vi "SPIM.vi"() -> ()   [LabVIEW 2015]
uses:
  Camera Properties.ctl
  Microscope Settings.ctl
  CameraState.ctl
  ModeEnum.ctl
  CameraControlTypeDef.ctl
  Stack Track.ctl
  Stack_State.ctl
  <vilib>/DAQmx/write.llb/DAQmx Write (Digital 1D Wfm NChan NSamp).vi
  <vilib>/DAQmx/write.llb/DAQmx Write (Analog 1D Wfm NChan NSamp).vi
  <vilib>/DAQmx/create/channels.llb/DAQmx Create Channel (DO-Digital Output).vi
  <vilib>/DAQmx/create/channels.llb/DAQmx Create Channel (AO-Voltage-Basic).vi
  <vilib>/Waveform/DWDTOps.llb/DWDT Append Digital Samples.vi
  <vilib>/Waveform/WDTOps.llb/WDT Append Waveforms DBL.vi
  <vilib>/Waveform/WDTOps.llb/WDT Number of Waveform Samples DBL.vi
  <vilib>/DAQmx/configure/timing.llb/DAQmx Timing (Sample Clock).vi
  <vilib>/Waveform/DWDTOps.llb/DWDT Uncompress Digital.vi
  <vilib>/DAQmx/miscellaneous.llb/DAQmx Fill In Error Info.vi
  <vilib>/vision/NI_Vision_Development_Module.lvlib
panel:
  in  "Tab Control":enum32{"Camera Settings", "Recording"}(tab)
  in  "Scans":dbl=1.0 min=0.0 max=10.0 step=0.05
  in  "?":bool
  in  "Microscope Settings":T1={"Mode"=enum."XY", "Slit"={"Scanning Mode"=12.0, "Slit Width /%"=5.0}, "Colour"=[{"Laser"=enum."561", "Filter"=4}], "Exposure/ms"=40.0, "Piezo Position /um"=0.0, "ROI"={"X"={"Start"=0.0, "Step"=1.0, "Range"=2048.0}, "Y"={"Start"=0.0, "Step"=1.0, "Range"=2048.0}, "Z "={"Start"=0.0, "Step"=1.0, "Range"=100.0}}, "Samples per millisecond"=100.0, "Relax/ms"=10.0, "Readout Direction"=2.0, "Trigger Source"=2.0, "Camera Delay /ms"=11.0, "Under Scan"=5.0} {"Under Scan" min=0.0 max=10.0 step=0.05; "ROI"."X"."Range" min=0.0 max=10.0 step=0.05; "ROI"."X"."Step" min=0.0 max=10.0 step=0.05; "ROI"."X"."Start" min=0.0 max=10.0 step=0.05; "ROI"."Y"."Range" min=0.0 max=10.0 step=0.05; "ROI"."Y"."Step" min=0.0 max=10.0 step=0.05; "ROI"."Y"."Start" min=0.0 max=10.0 step=0.05; "ROI"."Z"."Range" min=0.0 max=10.0 step=0.05; "ROI"."Z"."Step" min=0.0 max=10.0 step=0.05; "ROI"."Z"."Start" min=0.0 max=10.0 step=0.05; "Colour"."Filter" items=["Empty"=1, ""=2, ""=3, "561"=4, ""=5, "488"=6]; "Camera Delay /ms" min=0.0 max=10.0 step=0.05; "Trigger Source" items=["Internal"=1.0, "External"=2.0]; "Readout Direction" items=["Forward"=1.0, "Backward"=2.0]; "Slit"."Scanning Mode" items=["Full Frame"=1.0, "Slit Scanning"=12.0]; "Piezo Position /um" min=0.0 max=10.0 step=0.05}
  in  "Scan":bool
  in  "Scan Continuously":bool
  out "error IO":errorcluster
  in  "Advanced DCAM Controls":i32(listbox) caption="Multicolumn Listbox"
  in  "Properties":T2=4211904 items=["SENSOR MODE"=4212128, "CCD MODE"=4212384, "READOUT MODE"=4211872, "ACTIVE VIEW INDEX"=4343136, "BITS PER CHANNEL"=4342976, "IMAGE PIXEL TYPE"=4343296, "BINNING"=4215968, "EXPOSURE TIME"=2049184, "CONTRAST GAIN"=3163312, "CONTRAST OFFSET"=3163328, "LIGHT MODE"=2114720, "SENSITIVITY"=2114992, "PHOTON IMAGING MODE"=2115200, "HIGH DYNAMIC RANGE MODE"=3163360, "WHITE BALANCE"=3163568, "TEMPERATURE"=2115232, "TEMPERATURE TARGET"=2115264, "SENSOR COOLER FAN"=2115296, "LINEBUNDLE HEIGHT"=4212192, "MECHANICAL SHUTTER"=2115488, "BACK FOCUS POSITION"=8422304, "TRIGGER CONNECTOR"=1066432, "TRIGGER SOURCE"=1066144, "OUTPUT TRIGGER SOURCE"=1852576, "TRIGGER GLOBAL EXPOSURE"=2049680, "FIRST TRIGGER BEHAVIOR"=2049696, "CHANNEL SYNC"=1852352, "READOUT DIRECTION"=4211904, "PRE HSYNC COUNT"=1852704, "INTERNAL LINE SPEED"=4191408, "INTERNAL LINE INVERVAL"=4191424]
  out "appended path":path
  in  "Frames":i32
  in  "Imaging Folder":path=path "C:/_DATA/test/a.tif"
  in  "Multicolumn Listbox":i32(listbox)
  out "Image":T3(plugin-control)
  out "Histogram":T4(graph)
  in  "stop":bool
  in  "Record":bool
  in  "Signals Debugger":bool
  in  "Calibration":bool
  in  "MultiD Scan":bool
  in  "Stage Controller":bool
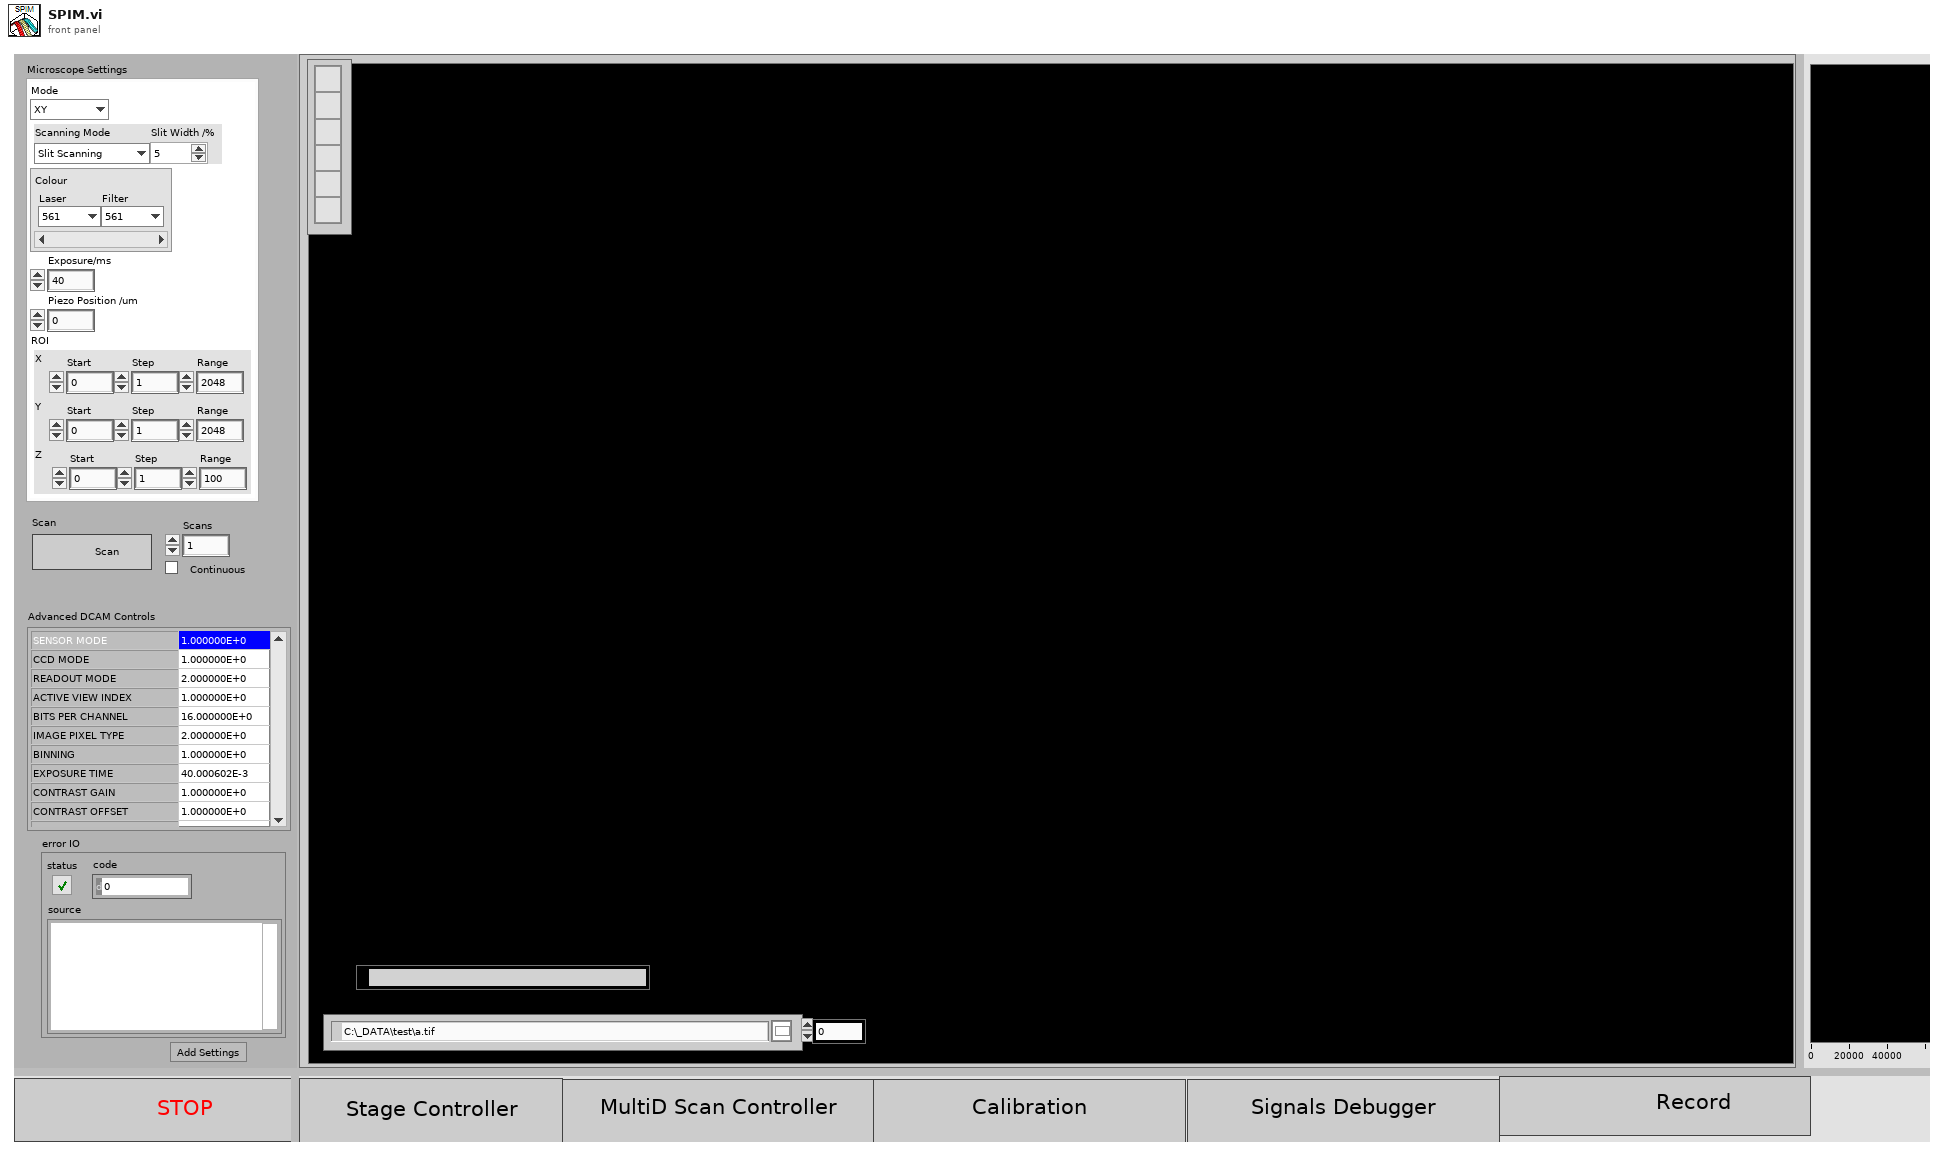
[diagram p1: front panel]
types:
  T1 = typedef "Microscope Settings.ctl" = cluster{"Mode":enum16{"X", "XY", "XYZ", "XYZT", "XYZC"}, "Slit":cluster{"Scanning Mode":dbl, "Slit Width /%":dbl}, "Colour":cluster{"Laser":enum16{"Brightfield", "445", "488", "561", "647"}, "Filter":u16}[], "Exposure/ms":dbl, "Piezo Position /um":dbl, "ROI":cluster{"X":cluster{"Start":dbl, "Step":dbl, "Range":dbl}, "Y":cluster{"Start":dbl, "Step":dbl, "Range":dbl}, "Z ":cluster{"Start":dbl, "Step":dbl, "Range":dbl}}, "Samples per millisecond":dbl, "Relax/ms":dbl, "Readout Direction":dbl, "Trigger Source":dbl, "Camera Delay /ms":dbl, "Under Scan":dbl}
  T2 = typedef "Camera Properties.ctl" = u32
  T3 = typedef "IMAQ Image.ctl" = refnum<image>
  T4 = cluster{"Starting Value":sgl, "Incremental Value":sgl, "Histogram":u32[]}
  T5 = cluster{"height":u32, "width":u32, "datatype":u32}
  T6 = typedef "CameraState.ctl" = enum16{"init", "active", "deinit"}
  T7 = typedef "ModeEnum.ctl" = enum16{"Idle", "generateWaves", "runWaves", "stop"}
  T8 = typedef "CameraControlTypeDef.ctl" = enum16{"Idle", "IntervalLineInt", "Ram Record", "HardDisk Record", "Disengage Update", "Update", "ROI", "Binning", "Scan Mode", "Trigger Mode", "Readout Mode", "Readout Direction", "Preview", "ROIWindow", "Trigger Source"}
  T9 = cluster{"Mode":u32, "Polarity":u32, "Times":u32, "Delay":dbl}
  T10 = typedef "Stack_State.ctl" = cluster{"State":T11, "Stack Number":i32, "Image":u16[][], "Stacks":i32}
  T11 = typedef "Stack Track.ctl" = enum16{"Idle", "Display", "Start Sequence", "Read Disk", "STOP", "Collecting", "End", "Save Image"}
  T12 = enum32{"Invalid", "Standard", "Closed", "Hidden", "Minimized", "Maximized"}
  T13 = typedef "Image Type" = u32
  T14 = cluster{"Analogue Out":waveform(dbl)[], "Digital Out":digitalwaveform[]}
  T15 = cluster{"State":T11, "Timeout":i32, "Data 16":u16[][], "Timeout":i32}
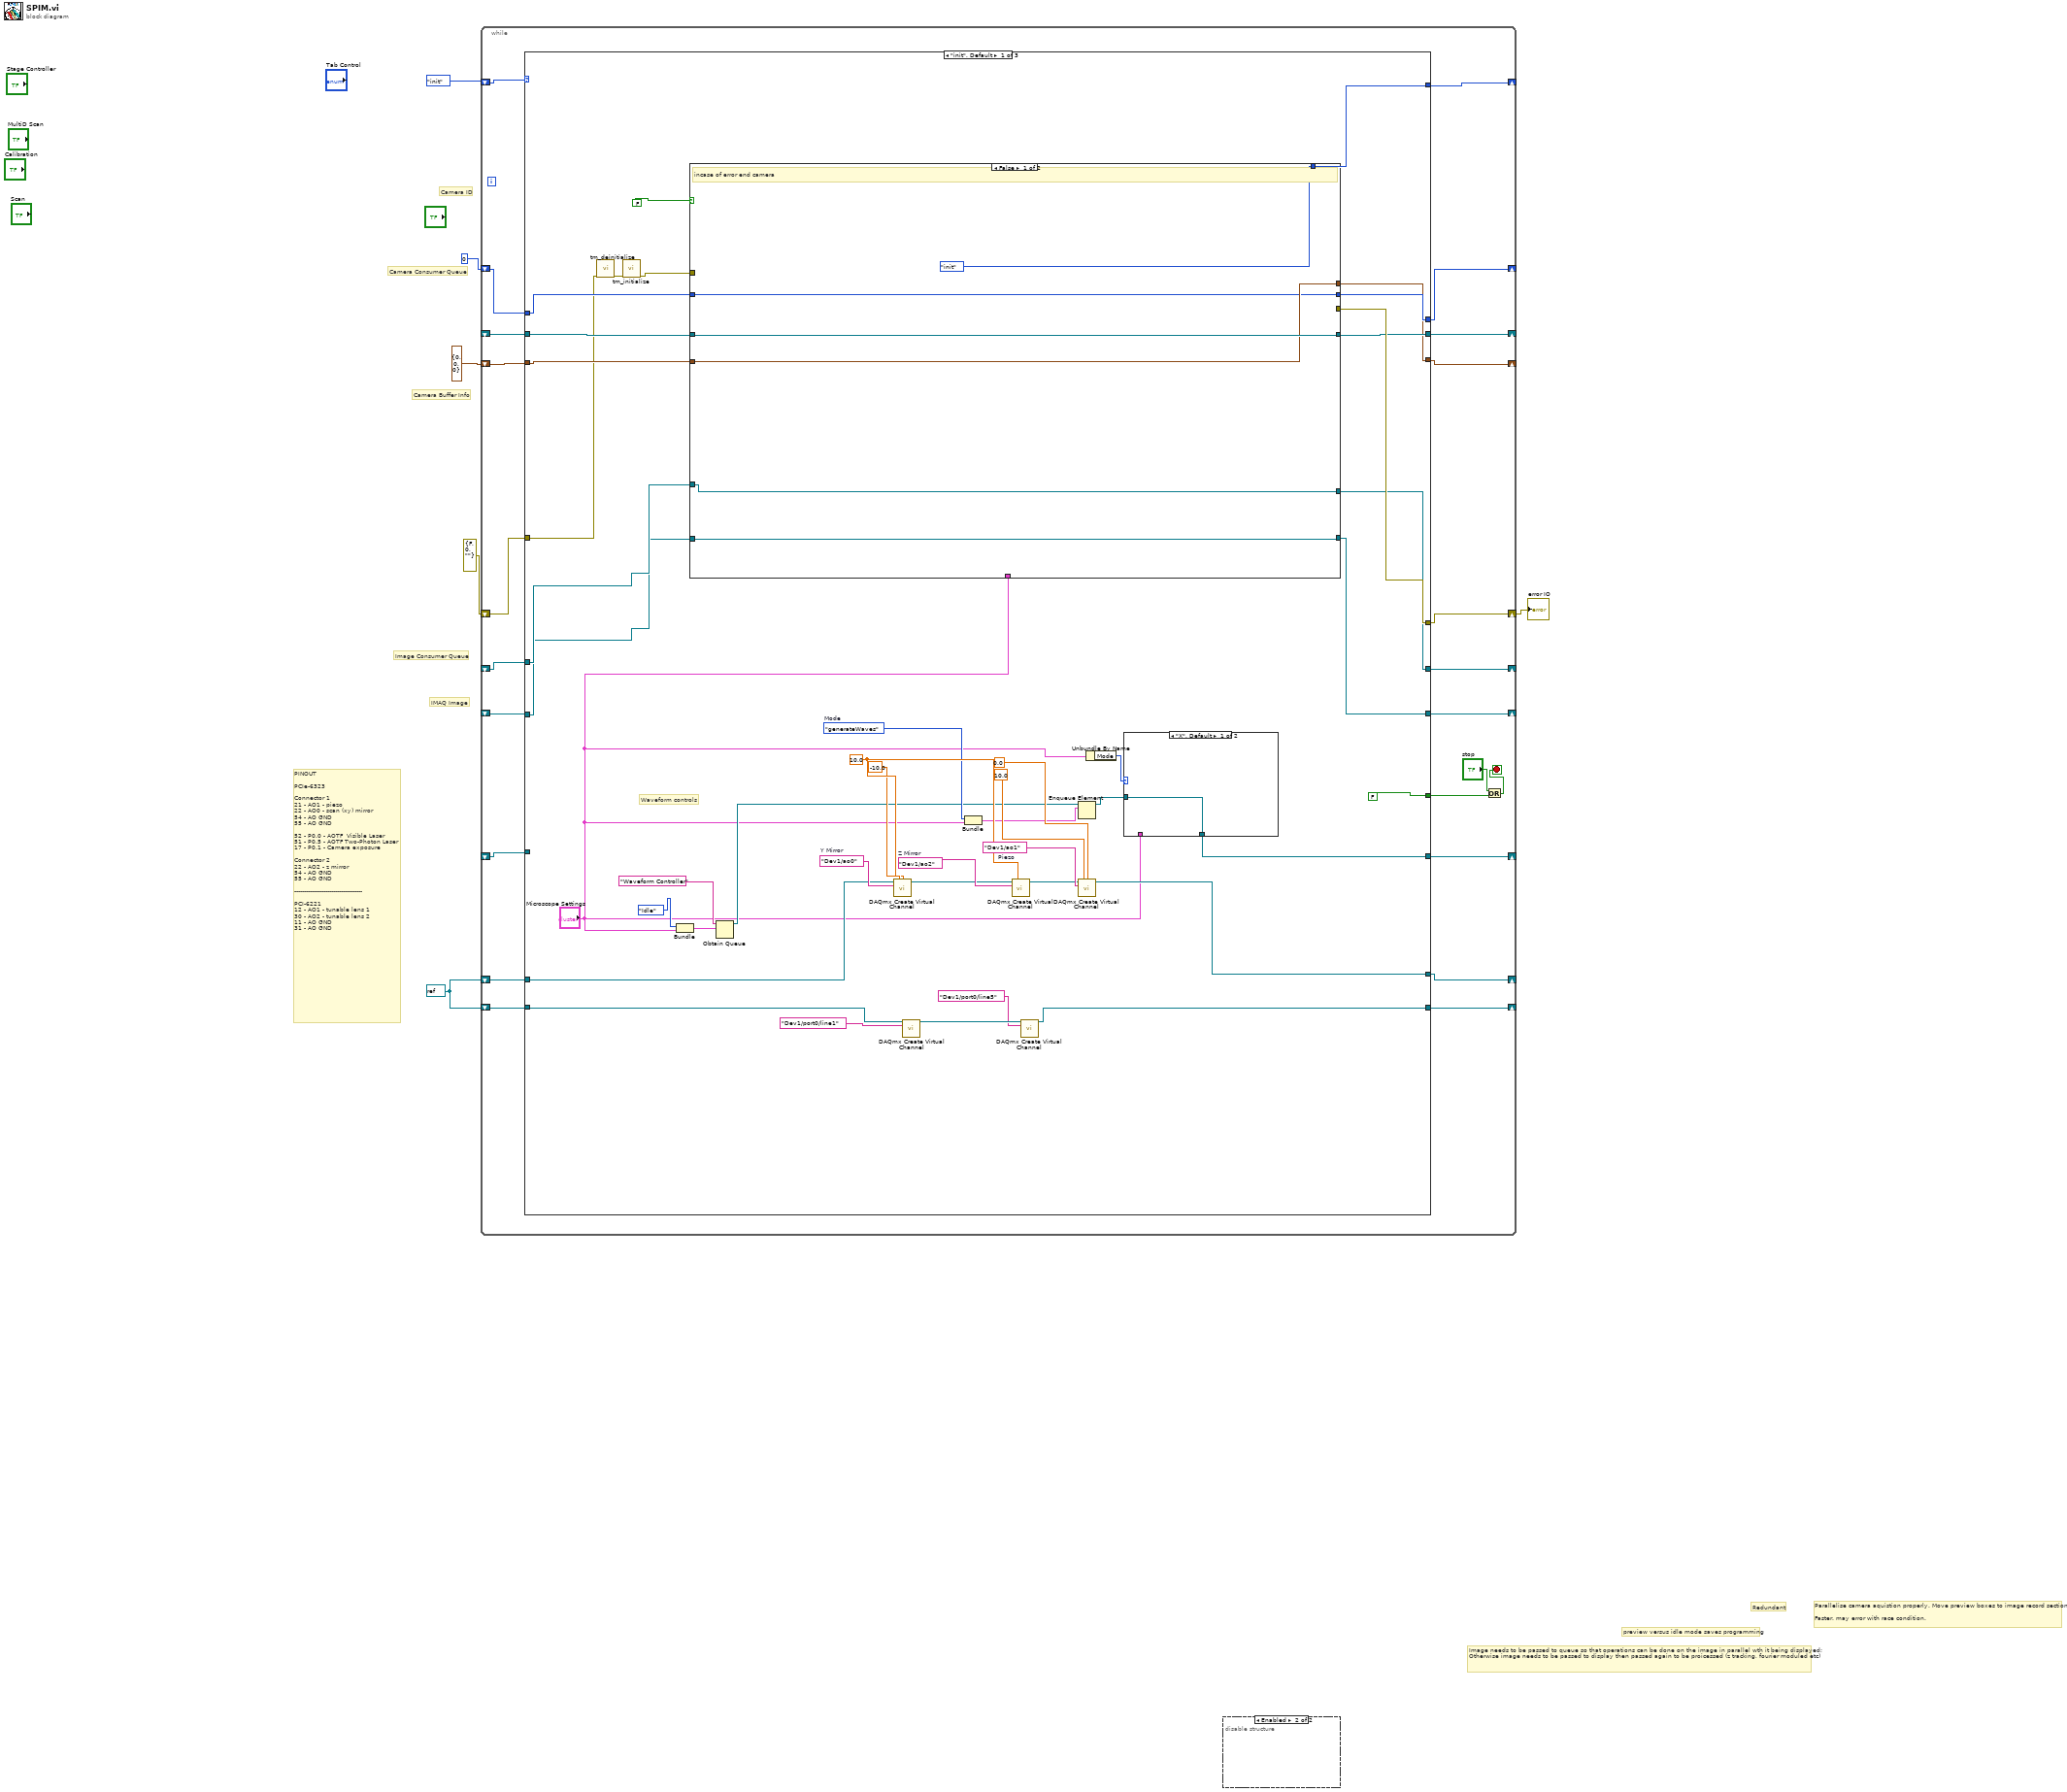
[diagram p0: block diagram]
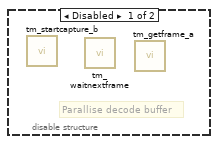
[diagram p2: hidden frame]
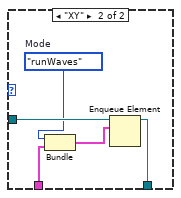
[diagram p3: hidden frame]
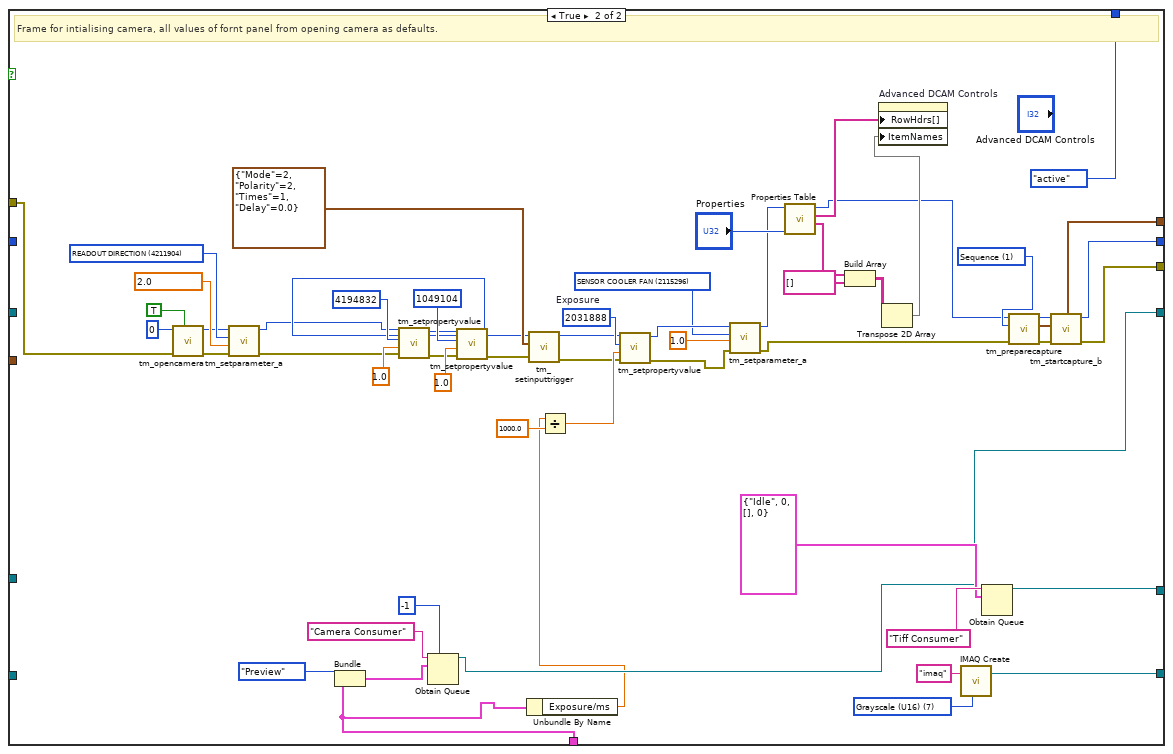
[diagram p4: hidden frame]
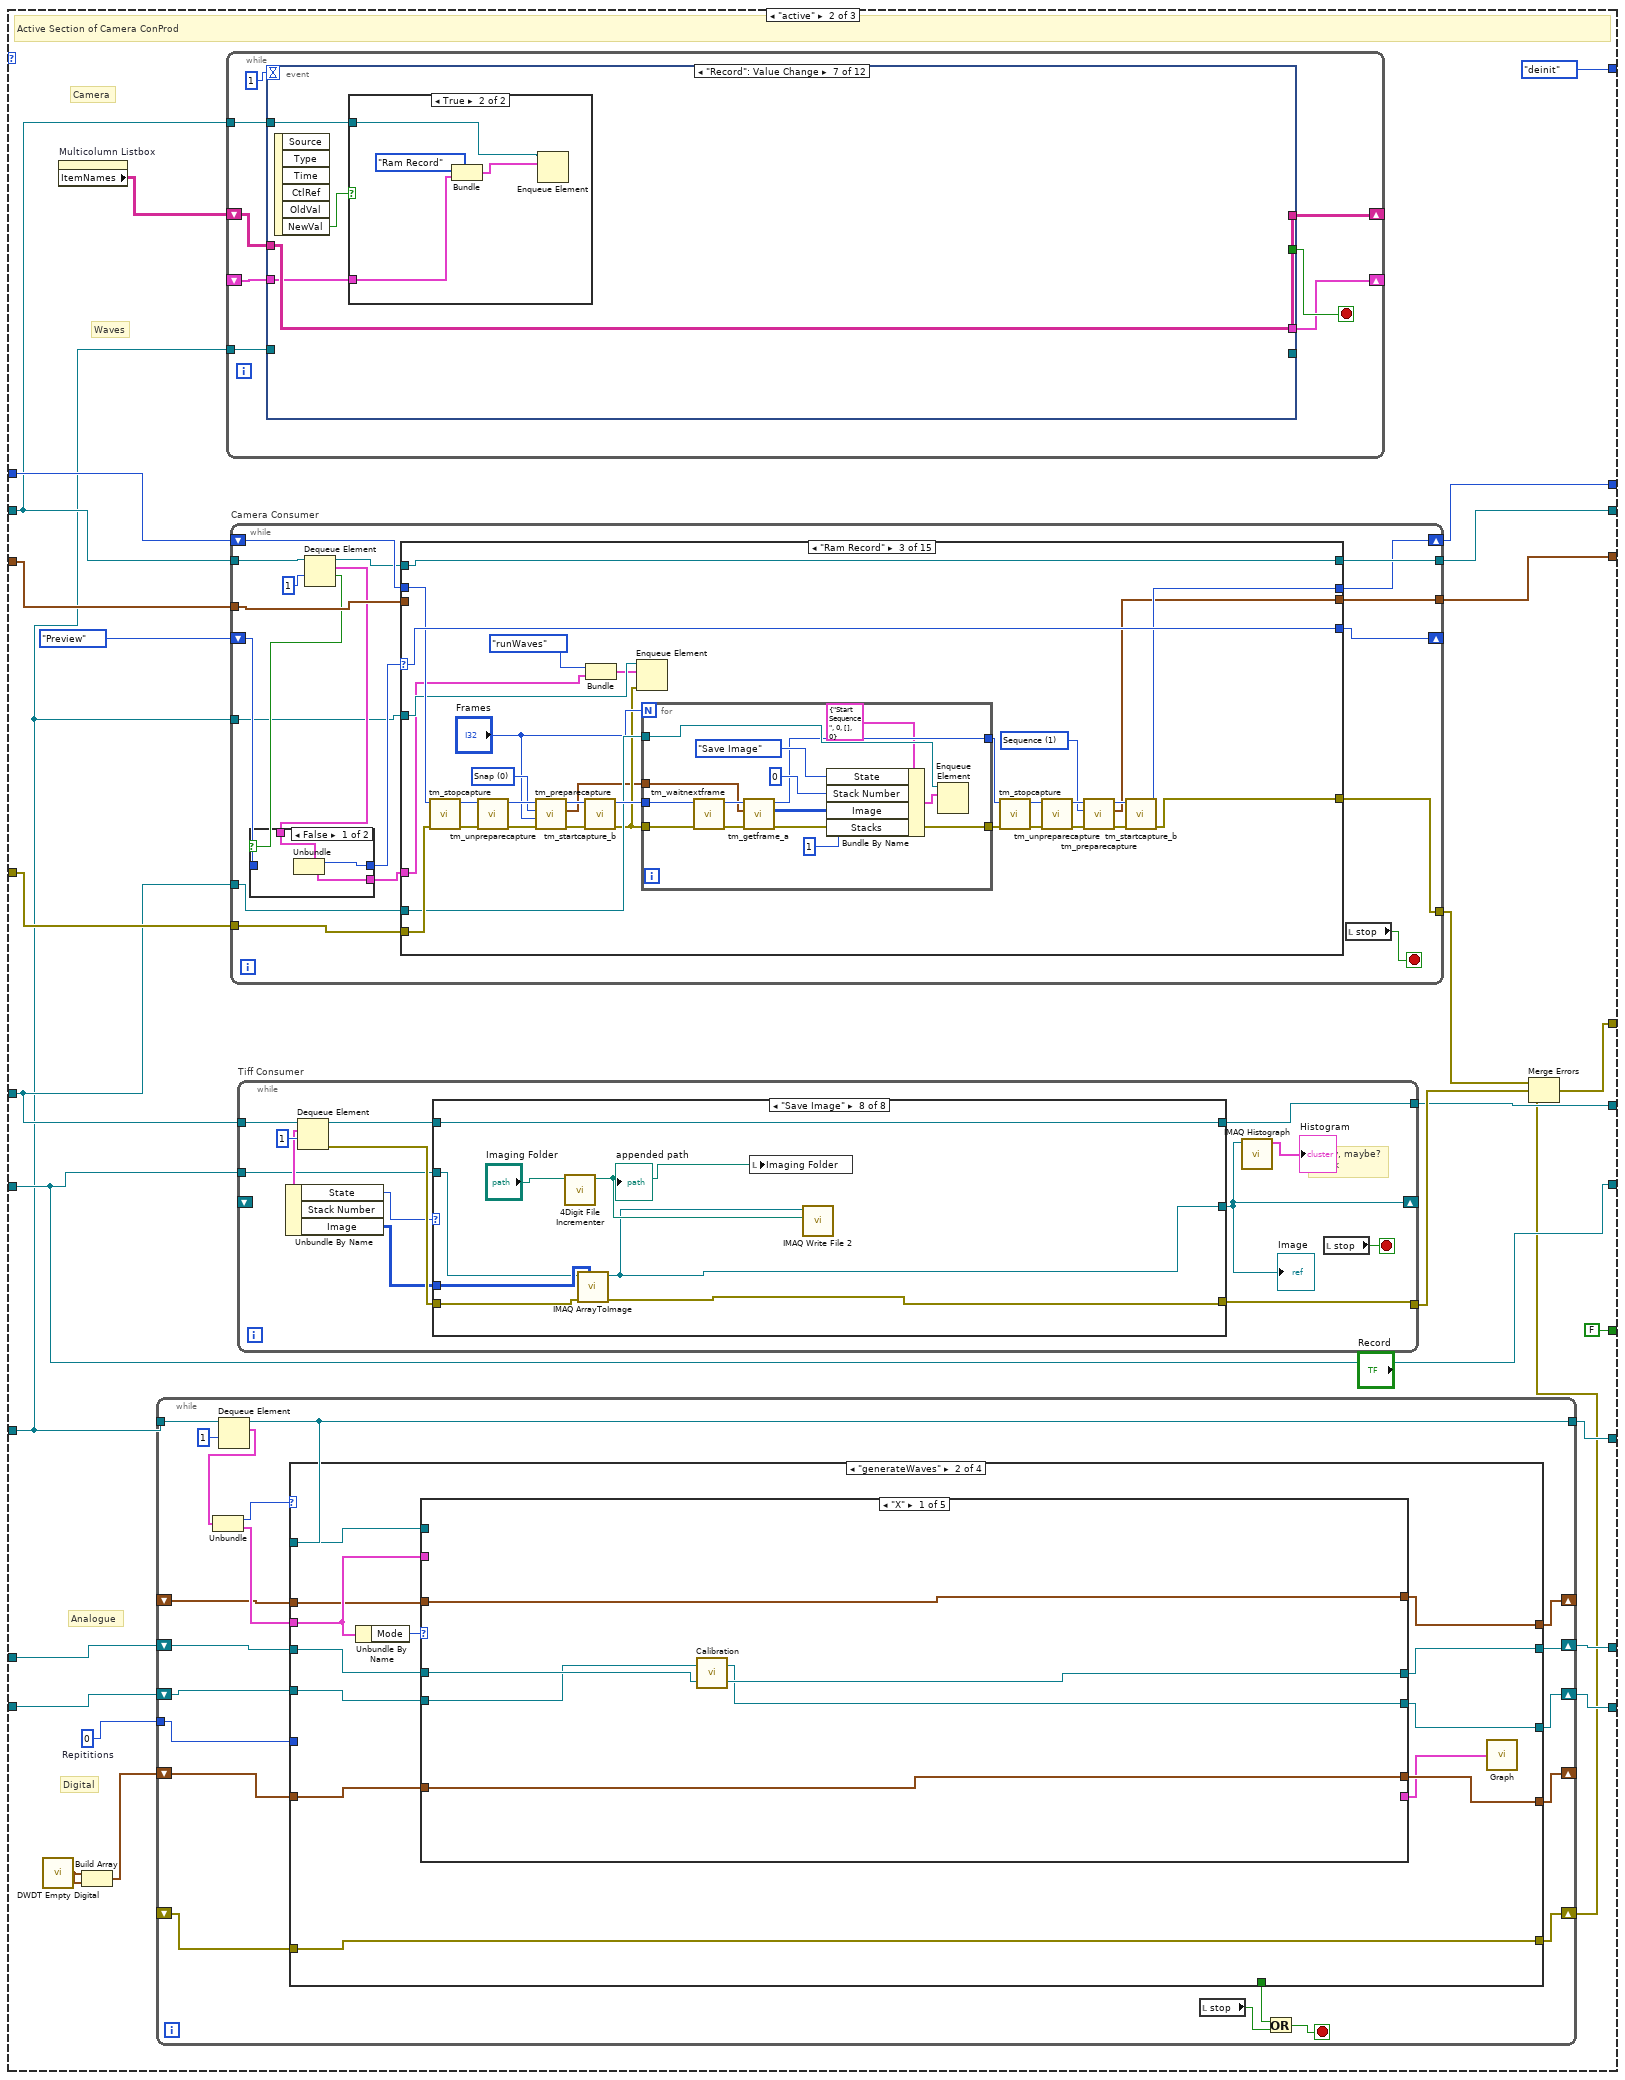
[diagram p5: hidden frame]
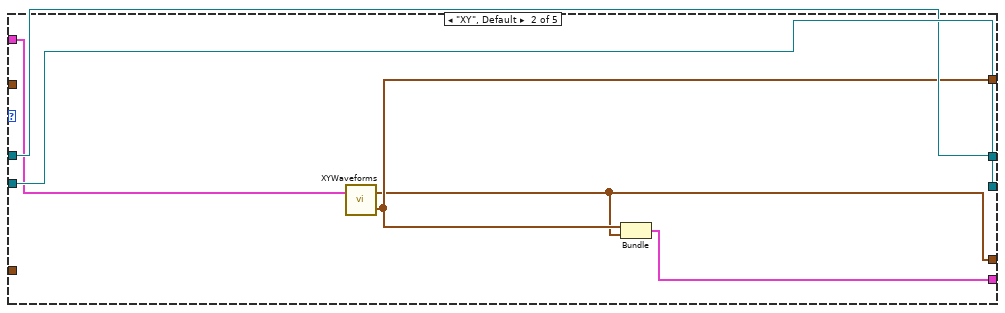
[diagram p7: hidden frame]
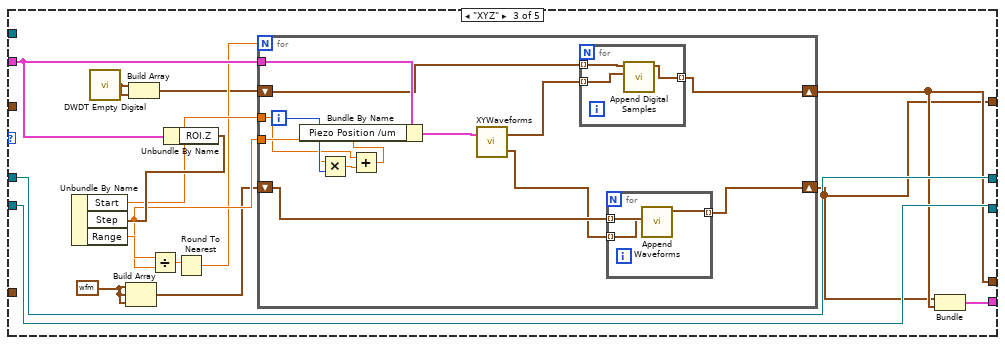
[diagram p8: hidden frame]
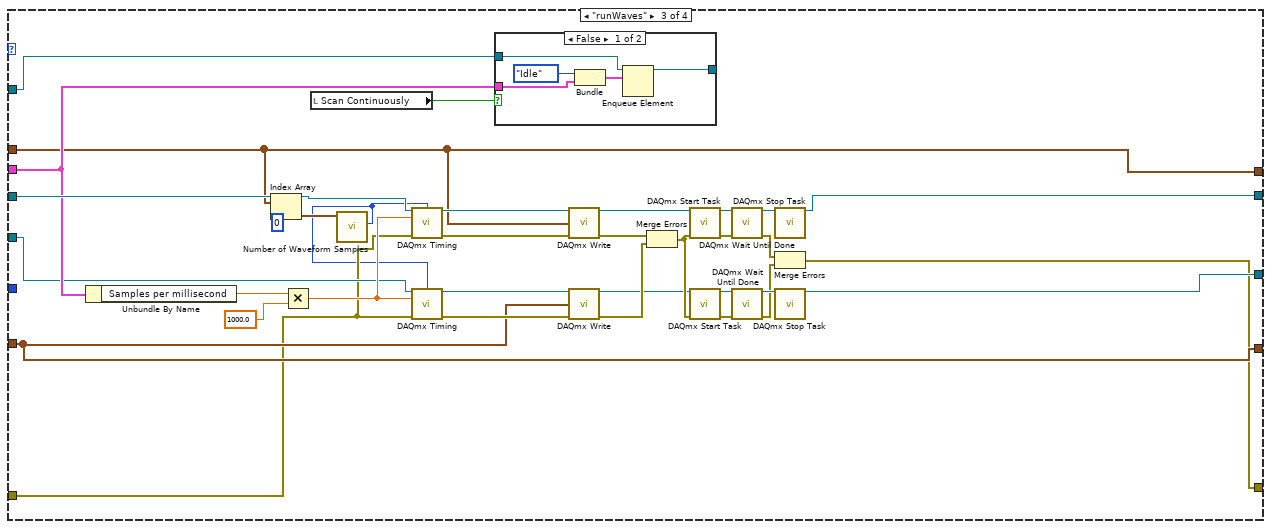
[diagram p11: hidden frame]
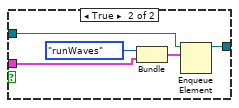
[diagram p12: hidden frame]
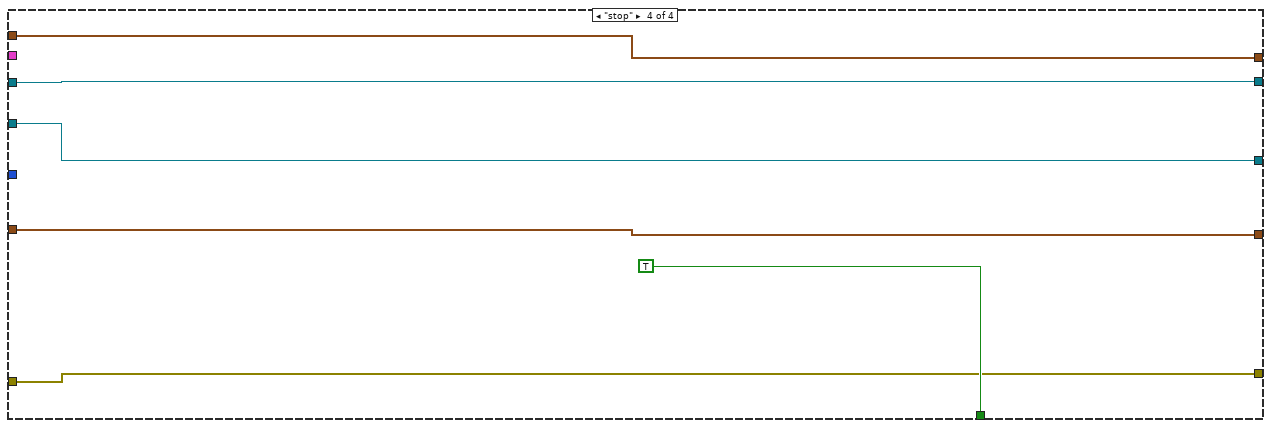
[diagram p13: hidden frame]
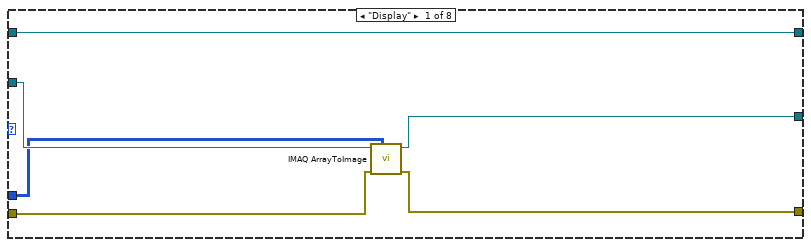
[diagram p14: hidden frame]
diagram:
  w3 = refnum<k21> refnum ("Mirror Z 2")
  # "PINOUT\n\nPCIe-6323\n\nConnector 1\n21 - AO1 - piezo\n22 - AO0 - scan (xy) mirror\n54 - AO GND\n55 - AO GND\n\n52 - P0.0 - AOTF  Visible Laser\n51 - P0.5 - AOTF Two-Photon Laser\n17 - P0.1 - Camera exposure\n\nConnector 2\n22 - AO2 - z mirror\n54 - AO GND\n55 - AO GND\n\n-----------------------------------\n\nPCI-6221\n12 - AO1 - tunable lens 1\n30 - AO2 - tunable lens 2\n11 - AO GND\n31 - AO GND"
  # "IMAQ Image"
  # "Camera Buffer Info"
  # "Image needs to be passed to queue so that operations can be done on the image in parallel wth it being displayed;\nOtherwise image needs to be passed to display then passed again to be proicessed (z tracking, fourier moduled etc)"
  # "preview versus idle mode saves programming"
  # "Parallelise camera aquistion properly. Move preview boxes to image record section.\n\nFaster. may error with race condition."
  # "Redundant"
  # "Image Consumer Queue"
  # "Camera Consumer Queue"
  # "Camera ID"
  n1 = while {
    shift-right: [w29] -> _
    shift-left: CameraState."init" -> [w28]
    shift-right: [w27] -> _
    shift-left: u32 0 ("Handle out") -> [w26]
    shift-right: [w25] -> w5
    shift-left: errorcluster {"status"=FALSE, "code"=0, "source"=""} ("error IO") -> [w24]
    shift-right: [w22] -> _
    shift-left: _ -> [w21]
    shift-right: [w23] -> _
    shift-left: _ -> [w20]
    shift-right: [w16] -> _
    shift-left: T5 {"height"=0, "width"=0, "datatype"=0} ("Buffer Info") -> [w15]
    shift-right: [w14] -> _
    shift-left: _ -> [w13]
    shift-right: [w12] -> _
    shift-left: w3 -> [w11]
    shift-right: [w9] -> _
    shift-left: w3 -> [w10]
    shift-right: [w8] -> _
    shift-left: _ -> [w7]
    stop <- w18 stop-if-true
    n2 = case shown="\"init\", Default" w28 {
      tunnel: [w71 CameraState."deinit" CameraState."init"] -> w29
      tunnel: [w70 w166 w697] -> w27
      tunnel: w26 -> [w48 w167 w697]
      tunnel: [w69 w165 w700] -> w25
      tunnel: w24 -> [w47 w159 w701]
      tunnel: [w68 w162 w684] -> w23
      tunnel: [w67 w161 w680] -> w22
      tunnel: w21 -> [w65 w154 w680]
      tunnel: w20 -> [w66 w152 w684]
      tunnel: [FALSE ("stop") FALSE ("stop") TRUE ("stop")] -> w17
      tunnel: [w63 w157 w694] -> w16
      tunnel: w15 -> [w62 w156 w694]
      tunnel: w13 -> [w60 w153 w693]
      tunnel: [w61 w153 w693] -> w14
      tunnel: w7 -> [_ w141 w679]
      tunnel: [w52 w145 w691] -> w12
      tunnel: w11 -> [w49 w148 w691]
      tunnel: w10 -> [w45 w147 w689]
      tunnel: [w40 w146 w689] -> w9
      tunnel: [w36 w144 w679] -> w8
      frame "init", Default {
        w44 = ModeEnum."generateWaves"  # Mode
        w55 = tag "Dev1/ao1"  # Piezo
        w56 = tag "Dev1/ao2"  # Z Mirror
        w57 = tag "Dev1/ao0"  # Y Mirror
        w59 = 10.0 ("maximum value")
        # "Waveform controls"
        n3 = call "tm_deinitialize.vi"("error in (no error)"=w47) -> ("error out"=w72:errorcluster)  [unwired: 10 in]
        n4 = call "tm_initialize.vi"("error in (no error)"=w72) -> ("error out"=w30:errorcluster)  [unwired: 7 in, 3 out]
        n5 = Bundle("Mode"=ModeEnum."Idle", "Microscope Settings"="Microscope Settings") -> (w42:cluster{"Mode":T7, "Microscope Settings":T1})  [unwired: 1 in]
        n6 = case shown="False" FALSE {
          tunnel: w30 -> [_ w105]
          tunnel: [CameraState."init" CameraState."active"] -> w71
          tunnel: [_ w136] -> w69
          tunnel: [w80 w134] -> w70
          tunnel: [w83 w124] -> w68
          tunnel: [w82 w131] -> w67
          tunnel: w66 -> [w83 _]
          tunnel: w65 -> [w82 _]
          tunnel: [w81 w129] -> w63
          tunnel: w62 -> [w81 _]
          tunnel: w48 -> [w80 _]
          tunnel: [w79 w126] -> w61
          tunnel: w60 -> [w79 _]
          tunnel: "Microscope Settings" -> [_ w92]
          frame False {
            # "incase of error end camera"
          }
          frame True {
            w102 = u32 2115296 items=["SENSOR MODE"=4212128, "CCD MODE"=4212384, "READOUT MODE"=4211872, "ACTIVE VIEW INDEX"=4343136, "BITS PER CHANNEL"=4342976, "IMAGE PIXEL TYPE"=4343296, "BINNING"=4215968, "EXPOSURE TIME"=2049184, "CONTRAST GAIN"=3163312, "CONTRAST OFFSET"=3163328, "LIGHT MODE"=2114720, "SENSITIVITY"=2114992, "PHOTON IMAGING MODE"=2115200, "HIGH DYNAMIC RANGE MODE"=3163360, "WHITE BALANCE"=3163568, "TEMPERATURE"=2115232, "TEMPERATURE TARGET"=2115264, "SENSOR COOLER FAN"=2115296, "LINEBUNDLE HEIGHT"=4212192, "MECHANICAL SHUTTER"=2115488, "BACK FOCUS POSITION"=8422304, "TRIGGER CONNECTOR"=1066432, "TRIGGER SOURCE"=1066144, "OUTPUT TRIGGER SOURCE"=1852576, "TRIGGER GLOBAL EXPOSURE"=2049680, "FIRST TRIGGER BEHAVIOR"=2049696, "CHANNEL SYNC"=1852352, "READOUT DIRECTION"=4211904, "PRE HSYNC COUNT"=1852704, "INTERNAL LINE SPEED"=4226000, "INTERNAL LINE INTERVAL"=4226016] ("Parameter")
            w111 = u32 2031888  # Exposure
            w122 = sgl 2.0 items=["Forward"=1.0, "Backward"=2.0] ("Readout Direction")
            w123 = u32 4211904 items=["SENSOR MODE"=4212128, "CCD MODE"=4212384, "READOUT MODE"=4211872, "ACTIVE VIEW INDEX"=4343136, "BITS PER CHANNEL"=4342976, "IMAGE PIXEL TYPE"=4343296, "BINNING"=4215968, "EXPOSURE TIME"=2049184, "CONTRAST GAIN"=3163312, "CONTRAST OFFSET"=3163328, "LIGHT MODE"=2114720, "SENSITIVITY"=2114992, "PHOTON IMAGING MODE"=2115200, "HIGH DYNAMIC RANGE MODE"=3163360, "WHITE BALANCE"=3163568, "TEMPERATURE"=2115232, "TEMPERATURE TARGET"=2115264, "SENSOR COOLER FAN"=2115296, "LINEBUNDLE HEIGHT"=4212192, "MECHANICAL SHUTTER"=2115488, "BACK FOCUS POSITION"=8422304, "TRIGGER CONNECTOR"=1066432, "TRIGGER SOURCE"=1066144, "OUTPUT TRIGGER SOURCE"=1852576, "TRIGGER GLOBAL EXPOSURE"=2049680, "FIRST TRIGGER BEHAVIOR"=2049696, "CHANNEL SYNC"=1852352, "READOUT DIRECTION"=4211904, "PRE HSYNC COUNT"=1852704, "INTERNAL LINE SPEED"=4226000, "INTERNAL LINE INTERVAL"=4226016] ("Parameter")
            w128 = T13 7 items=["Grayscale (U8)", "Grayscale (I16)", "Grayscale (SGL)", "Complex (CSG)", "RGB (U32)", "HSL (U32)", "RGB (U64)", "Grayscale (U16)"] ("Image Type")
            w138 = 1 items=["Snap", "Sequence"] ("Capture mode")
            # "Frame for intialising camera, all values of fornt panel from opening camera as defaults."
            n7 = call "tm_opencamera.vi"("Force Open"=TRUE, "error in (no error)"=w105, "Camera Index"=u32 0) -> ("error out"=w120:errorcluster, "Handle out"=w121:u32)  [unwired: 6 in, 1 out]
            n8 = call "tm_setparameter_a.vi"("error in (no error)"=w120, "Value in"=w122, "Parameter"=w123, "Handle in"=w121) -> ("error out"=w90:errorcluster, "Handle out"=w112:u32)  [unwired: 6 in]
            n9 = Bundle("Enum"=CameraControlTypeDef."Preview", "Microscope Settings"=w92) -> (w106:cluster{"Enum":T8, "Microscope Settings":T1})  [unwired: 1 in]
            n10 = call "tm_setpropertyvalue.vi"("error in (no error)"=w90, "Value in"=sgl 1.0, "Property ID"=u32 4194832, "Handle in"=w112) -> ("error out"=w89:errorcluster, "Handle out"=w115:u32)  [unwired: 6 in]
            n11 = Obtain Queue(max queue size (-1, unlimited)=-1, name (unnamed)="Camera Consumer", element data type=w106) -> (queue out=w124:refnum<queue>)  [unwired: 2 in, 2 out]
            n12 = call "tm_setpropertyvalue.vi"("error in (no error)"=w89, "Value in"=sgl 1.0, "Property ID"=u32 1049104, "Handle in"=w115) -> ("error out"=w88:errorcluster, "Handle out"=w113:u32)  [unwired: 6 in]
            n13 = Unbundle By Name(w92) -> ("Exposure/ms"=w91:dbl)
            n14 = call <userlib>:"tm_setinputtrigger.vi"("error in (no error)"=w88, "Parameters"=T9 {"Mode"=2, "Polarity"=2, "Times"=1, "Delay"=0.0}, "Handle in"=w113) -> ("error out"=w87:errorcluster, "Handle out"=w110:u32)  [unwired: 7 in]
            n15 = Divide(x=w91, y=sgl 1000.0) -> (x/y=w108:dbl)
            n16 = call "tm_setpropertyvalue.vi"("error in (no error)"=w87, "Value in"=w108, "Property ID"=w111, "Handle in"=w110) -> ("error out"=w86:errorcluster, "Handle out"=w103:u32)  [unwired: 6 in]
            n17 = call "tm_setparameter_a.vi"("error in (no error)"=w86, "Value in"=1.0, "Parameter"=w102, "Handle in"=w103) -> ("error out"=w85:errorcluster, "Handle out"=w94:u32)  [unwired: 6 in]
            n18 = call "Properties Table.vi"("Properties"="Properties", "Handle In"=w94) -> ("Value Stirngs Out"=w98:string[], "Row Headers"=w99:string[], "Handle Out"=w93:u32)  [unwired: 3 in, 1 out]
            n19 = Build Array(w98, string[] [] ("element")) -> (w96:string[][])
            n20 = Transpose 2D Array(2D array=w96) -> (transposed array=w95:string[][])
            n21 = property on="Advanced DCAM Controls" class="MCListbox (strict)"("RowHdrs[]"=w99, "ItemNames"=w95) -> ()  [unwired: 2 in, 2 out]
            n22 = call "IMAQ Create"("Image Name"="imaq", "Image Type"=w128) -> ("New Image"=w126:T3)  [unwired: 3 in, 1 out]
            n23 = Obtain Queue(name (unnamed)="Tiff Consumer", element data type=T10 {"State"=enum."Idle", "Stack Number"=0, "Image"=[], "Stacks"=0} ("input cluster")) -> (queue out=w131:refnum<queue>)  [unwired: 3 in, 2 out]
            n24 = call "tm_preparecapture.vi"("error in (no error)"=w85, "Capture mode"=w138, "Handle in"=w93) -> ("error out"=w137:errorcluster, "Buffer Info"=w129:T5, "Handle out"=w135:u32)  [unwired: 5 in, 1 out]
            n25 = call "tm_startcapture_b.vi"("error in (no error)"=w137, "Handle in"=w135) -> ("error out"=w136:errorcluster, "Handle out"=w134:u32)  [unwired: 8 in]
          }
        }
        n26 = Obtain Queue(name (unnamed)="Waveform Controller", element data type=w42) -> (queue out=w41:refnum<queue>)  [unwired: 3 in, 2 out]
        n27 = call-poly <vilib>:"DAQmx Create Virtual Channel.vi"("task in"=w49, "maximum value"=w59, "minimum value"=-10.0, "physical channels"=w57) -> ("task out"=w51:refnum<k21>)  [unwired: 10 in, 1 out]
        n28 = call-poly <vilib>:"DAQmx Create Virtual Channel.vi"("task in"=w45, "lines"=tag "Dev1/port0/line1") -> ("task out"=w46:refnum<k21>)  [unwired: 12 in, 1 out]
        n29 = Bundle("Mode"=w44, "Microscope Settings"="Microscope Settings") -> (w33:cluster{"Mode":T7, "Microscope Settings":T1})  [unwired: 1 in]
        n30 = call-poly <vilib>:"DAQmx Create Virtual Channel.vi"("task in"=w51, "maximum value"=w59, "physical channels"=w56) -> ("task out"=w50:refnum<k21>)  [unwired: 11 in, 1 out]
        n31 = call-poly <vilib>:"DAQmx Create Virtual Channel.vi"("task in"=w46, "lines"=tag "Dev1/port0/line5") -> ("task out"=w40:refnum<k21>)  [unwired: 12 in, 1 out]
        n32 = Enqueue Element(queue=w41, element=w33) -> (queue out=w37:refnum<queue>)  [unwired: 2 in, 2 out]
        n33 = call-poly <vilib>:"DAQmx Create Virtual Channel.vi"("task in"=w50, "maximum value"=10.0 ("minimum value"), "minimum value"=0.0 ("maximum value"), "physical channels"=w55) -> ("task out"=w52:refnum<k21>)  [unwired: 10 in, 1 out]
        n34 = Unbundle By Name("Microscope Settings") -> ("Mode"=w32:enum16{"X", "XY", "XYZ", "XYZT", "XYZC"})
        n35 = case shown="\"X\", Default" w32 {
          tunnel: w37 -> [w73 w78]
          tunnel: [w73 w76] -> w36
          tunnel: "Microscope Settings" -> [_ w75]
          frame "X", Default {
          }
          frame "XY" {
            w74 = ModeEnum."runWaves"  # Mode
            n36 = Bundle("Mode"=w74, "Microscope Settings"=w75) -> (w77:cluster{"Mode":T7, "Microscope Settings":T1})  [unwired: 1 in]
            n37 = Enqueue Element(queue=w78, element=w77) -> (queue out=w76:refnum<queue>)  [unwired: 2 in, 2 out]
          }
        }
      }
      frame "active" {
        w151 = 0  # Repititions
        # "Waves"
        # "Camera"
        # "Digital"
        # "Analogue"
        # "Active Section of Camera ConProd"
        n38 = call <vilib>:"DWDT Empty Digital.vi"() -> ("digital waveform out"=w149:digitalwaveform)  [unwired: 5 in]
        n39 = property on="Multicolumn Listbox" class="MCListbox (strict)"() -> ("ItemNames"=w142:string[][])  [unwired: 2 in, 2 out]
        n40 = Build Array(w149, w149) -> (w150:digitalwaveform[])
        n41 = while {
          tunnel: w141 -> [w187]
          shift-right: [w183] -> _
          shift-left: _ -> [w182]
          tunnel: w151 -> [w181]
          shift-right: [w177] -> w145
          shift-left: w148 -> [w176]
          shift-right: [w180] -> _
          shift-left: w150 -> [w179]
          shift-right: [w175] -> w146
          shift-left: w147 -> [w174]
          tunnel: [w173] -> w144
          shift-right: [w172] -> w143
          shift-left: _ -> [w171]
          stop <- w168 stop-if-true
          n42 = Dequeue Element(queue=w187, timeout in ms (-1)=1) -> (queue out=w173:refnum<queue>, element=w186:cluster{"Mode":T7, "Microscope Settings":T1})  [unwired: 1 in, 2 out]
          n43 = Unbundle(w186) -> ("Mode"=w185:T7, "Microscope Settings"=w184:T1)
          n44 = case shown="\"generateWaves\"" w185 {
            tunnel: [_ _ _ TRUE] -> w170
            tunnel: w184 -> [_ w204 w289 _]
            tunnel: [w192 w205 w288 w310] -> w183
            tunnel: w182 -> [w192 w196 w288 w310]
            tunnel: w181 -> [_ _ _ _]
            tunnel: w173 -> [_ w195 w290 _]
            tunnel: [w189 w200 w268 w309] -> w175
            tunnel: [w190 w198 w283 w308] -> w177
            tunnel: w176 -> [w190 w197 w291 w308]
            tunnel: [w191 w203 w270 w307] -> w180
            tunnel: w179 -> [w191 w202 w270 w307]
            tunnel: w174 -> [w189 w201 w279 w309]
            tunnel: [w188 w194 w265 w305] -> w172
            tunnel: w171 -> [w188 w194 w264 w305]
            frame "Idle", Default {
            }
            frame "generateWaves" {
              n45 = Unbundle By Name(w204) -> ("Mode"=w199:enum16{"X", "XY", "XYZ", "XYZT", "XYZC"})
              n46 = case shown="\"X\"" w199 {
                tunnel: [w211 w214 w222 w256 w260] -> w205
                tunnel: w204 -> [_ w215 w233 _ _]
                tunnel: [w210 w213 w226 w253 w257] -> w203
                tunnel: w202 -> [w210 _ _ w253 w257]
                tunnel: w201 -> [w207 w217 w227 w254 w258]
                tunnel: [w206 w217 w227 w254 w258] -> w200
                tunnel: [w209 w216 w228 w255 w259] -> w198
                tunnel: w197 -> [w208 w216 w228 w255 w259]
                tunnel: w196 -> [w211 _ _ w256 w260]
                tunnel: w195 -> [_ _ _ _ _]
                tunnel: [_ w212 w223 _ _] -> w193
                frame "X" {
                  n47 = call "Calibration.vi"("Analogue In"=w208, "Digital In"=w207) -> ("Analogue In Out"=w209:refnum<k21>, "Digital Out"=w206:refnum<k21>)
                }
                frame "XY", Default {
                  n48 = call "XYWaveforms.vi"("Microscope Settings"=w215) -> ("Analogue Out"=w214:waveform(dbl)[], "Digital Out"=w213:digitalwaveform[])  [unwired: 1 in]
                  n49 = Bundle("Analogue Out"=w214, "Digital Out"=w213) -> (w212:T14)  [unwired: 1 in]
                }
                frame "XYZ" {
                  w218 = waveform(dbl) {"t0"=timestamp(0 s since 1904-01-01), "dt"=1.0, "Y"=[]} ("Waveform")
                  n50 = call <vilib>:"DWDT Empty Digital.vi"() -> ("digital waveform out"=w221:digitalwaveform)  [unwired: 5 in]
                  n51 = Build Array(w218, w218, w218) -> (w219:waveform(dbl)[])
                  n52 = Build Array(w221, w221) -> (w220:digitalwaveform[])
                  n53 = Unbundle By Name(w233) -> ("ROI.Z"=w232:cluster{"Start":dbl, "Step":dbl, "Range":dbl})
                  n54 = Unbundle By Name(w232) -> ("Start"=w231:dbl, "Step"=w229:dbl, "Range"=w230:dbl)
                  n55 = Divide(x=w230, y=w229) -> (x/y=w225:dbl)
                  n56 = Round To Nearest(number=w225) -> (nearest integer value=w224:dbl)
                  n57 = for {
                    N: w224 -> [_]
                    tunnel: w233 -> [w246]
                    tunnel: w229 -> [w242]
                    tunnel: w231 -> [w241]
                    shift-right: [w237] -> w222
                    shift-left: w219 -> [w239]
                    shift-right: [w235] -> w226
                    shift-left: w220 -> [w234]
                    i -> [w243]
                    n58 = Multiply(x=w242, y=w243) -> (x*y=w244:dbl)
                    n59 = Add(x=w241, y=w244) -> (x+y=w240:dbl)
                    n60 = Bundle By Name(cluster=w246, "Piezo Position /um"=w240) -> (w245:T1)
                    n61 = call "XYWaveforms.vi"("Microscope Settings"=w245) -> ("Analogue Out"=w238:waveform(dbl)[], "Digital Out"=w236:digitalwaveform[])  [unwired: 1 in]
                    n62 = for {
                      tunnel: w236 -> [w248] mode=indexing
                      tunnel: w234 -> [w249] mode=indexing
                      tunnel: [w247] -> w235 mode=indexing
                      n63 = call-poly <vilib>:"Append Digital Samples.vi"("digital waveform B"=w248, "digital waveform A"=w249) -> ("digital waveform out"=w247:digitalwaveform)  [unwired: 8 in, 1 out]
                    }
                    n64 = for {
                      tunnel: w238 -> [w251] mode=indexing
                      tunnel: w239 -> [w252] mode=indexing
                      tunnel: [w250] -> w237 mode=indexing
                      n65 = call-poly <vilib>:"Append Waveforms.vi"("waveform B"=w251, "waveform A"=w252) -> ("waveform out"=w250:waveform(dbl))  [unwired: 8 in, 1 out]
                    }
                  }
                  n66 = Bundle(w222, w226) -> (w223:cluster{waveform(dbl)[], digitalwaveform[]})  [unwired: 1 in]
                }
                frame "XYZT" {
                }
                frame "XYZC" {
                }
              }
              n67 = call "Graph.vi"("Cluster"=w193) -> ()
            }
            frame "runWaves" {
              n68 = Unbundle By Name(w289) -> ("Samples per millisecond"=w261:dbl)
              n69 = Index Array(array=w288, index=0) -> (element=w286:waveform(dbl))
              n70 = Multiply(x=w261, y=1000.0) -> (x*y=w281:dbl)
              n71 = local read "Scan Continuously"() -> (w282:bool)
              n72 = call-poly <vilib>:"Number of Waveform Samples.vi"("waveform in"=w286) -> ("number of samples"=w262:i32)  [unwired: 8 in, 2 out]
              n73 = call-poly <vilib>:"DAQmx Timing.vi"("task/channels in"=w291, "samples per channel"=w262, "rate"=w281, "error in"=w264) -> ("task out"=w294:refnum<k21>, "error out"=w285:errorcluster)  [unwired: 10 in]
              n74 = call-poly <vilib>:"DAQmx Timing.vi"("task/channels in"=w279, "samples per channel"=w262, "rate"=w281, "error in"=w264) -> ("task out"=w280:refnum<k21>, "error out"=w277:errorcluster)  [unwired: 10 in]
              n75 = case shown="False" w282 {
                tunnel: w290 -> [w296 w304]
                tunnel: [w297 w303] -> _
                tunnel: w289 -> [w298 w302]
                frame False {
                  n76 = Bundle("Mode"=ModeEnum."Idle", "Microscope Settings"=w298) -> (w299:cluster{"Mode":T7, "Microscope Settings":T1})  [unwired: 1 in]
                  n77 = Enqueue Element(queue=w296, element=w299) -> (queue out=w297:refnum<queue>)  [unwired: 2 in, 2 out]
                }
                frame True {
                  n78 = Bundle("Mode"=ModeEnum."runWaves", "Microscope Settings"=w302) -> (w301:cluster{"Mode":T7, "Microscope Settings":T1})  [unwired: 1 in]
                  n79 = Enqueue Element(queue=w304, element=w301) -> (queue out=w303:refnum<queue>)  [unwired: 2 in, 2 out]
                }
              }
              n80 = call-poly <vilib>:"DAQmx Write.vi"("task/channels in"=w294, "data"=w288, "error in"=w285) -> ("task out"=w272:refnum<k21>, "error out"=w275:errorcluster)  [unwired: 10 in, 1 out]
              n81 = call-poly <vilib>:"DAQmx Write.vi"("task/channels in"=w280, "data"=w270, "error in"=w277) -> ("task out"=w271:refnum<k21>, "error out"=w274:errorcluster)  [unwired: 10 in, 1 out]
              n82 = Merge Errors(w275, w274) -> (w273:errorcluster)
              n83 = call <vilib>:"DAQmx Start Task.vi"("task/channels in"=w272, "error in"=w273) -> ("task out"=w293:refnum<k21>, "error out"=w292:errorcluster)  [unwired: 12 in]
              n84 = call <vilib>:"DAQmx Start Task.vi"("task/channels in"=w271, "error in"=w273) -> ("task out"=w278:refnum<k21>, "error out"=w276:errorcluster)  [unwired: 12 in]
              n85 = call <vilib>:"DAQmx Wait Until Done.vi"("task/channels in"=w293, "error in"=w292) -> ("task out"=w284:refnum<k21>, "error out"=w267:errorcluster)  [unwired: 12 in]
              n86 = call <vilib>:"DAQmx Wait Until Done.vi"("task/channels in"=w278, "error in"=w276) -> ("task out"=w269:refnum<k21>, "error out"=w266:errorcluster)  [unwired: 12 in]
              n87 = call <vilib>:"DAQmx Stop Task.vi"("task/channels in"=w284) -> ("task out"=w283:refnum<k21>)  [unwired: 13 in, 1 out]
              n88 = Merge Errors(w267, w266) -> (w265:errorcluster)
              n89 = call <vilib>:"DAQmx Stop Task.vi"("task/channels in"=w269) -> ("task out"=w268:refnum<k21>)  [unwired: 13 in, 1 out]
            }
            frame "stop" {
            }
          }
          n90 = local read "stop"() -> (w169:bool)
          n91 = Or(x=w170, y=w169) -> (x .or. y?=w168:bool)
        }
        n92 = while {
          tunnel: w152 -> [w592]
          shift-right: [w591] -> _
          shift-left: _ -> [w590]
          tunnel: w141 -> [w588]
          shift-right: [w587] -> _
          shift-left: w142 -> [w586]
          stop <- w593 stop-if-true
          n93 = event shown="[6] \"Record\": Value Change" {
            selector: _ -> [_ _ _ _ _ _ _ _ _ _ _ _]
            dyn-events: _ -> [_ _ _ _ _ _ _ _ _ _ _ _]
            timeout: 1 -> [_ _ _ _ _ _ _ _ _ _ _ _]
            tunnel: [w602 _ _ _ _ _ _ _ _ _ _ _] -> w593
            tunnel: w592 -> [w597 _ w616 w621 w628 _ w638 _ w651 _ _ _]
            tunnel: [w595 _ w610 w619 _ _ _ _ _ _ _ w678] -> w591
            tunnel: w590 -> [w595 w608 w610 w619 w624 w631 w637 w646 w652 _ w666 _]
            tunnel: [_ _ _ w620 _ _ _ _ _ _ w665 _] -> _
            tunnel: w588 -> [w596 _ w615 w620 w625 w632 _ w645 w650 _ w664 _]
            tunnel: [w594 w603 w609 w617 w627 w635 w639 w644 w649 w658 w662 w677] -> w587
            tunnel: w586 -> [w594 w605 w609 w617 w627 w635 w639 w644 w649 w658 w662 w677]
            event "stop": Value Change {
              w600 = ModeEnum."stop"  # Mode
              n94 = event-data() -> ()  [unwired: 1 in, 6 out]
              n95 = Bundle("Enum"=CameraControlTypeDef."Idle", "Value"=w595) -> (w598:cluster{"Enum":T8, "Value":T1})  [unwired: 1 in]
              n96 = Bundle("Mode"=w600, "Value"=w595) -> (w599:cluster{"Mode":T7, "Value":T1})  [unwired: 1 in]
              n97 = Enqueue Element(queue=w597, element=w598) -> ()  [unwired: 2 in, 3 out]
              n98 = Enqueue Element(queue=w596, element=w599) -> ()  [unwired: 2 in, 3 out]
              n99 = local read "stop"() -> (w602:bool)
            }
            event Value Change {
              n100 = event-data() -> ()  [unwired: 1 in, 6 out]
              n101 = Flatten To XML(anything=w608) -> (xml string=w607:string)
              n102 = Build Array("Experiment 1" ("element"), w607) -> (w604:string[])
              n103 = Build Array (concatenate)(w605, w604) -> (w603:string[][])
              n104 = property on="Multicolumn Listbox" class="MCListbox (strict)"("ItemNames"=w603) -> ()  [unwired: 2 in, 2 out]
            }
            event Value Change {
              w613 = ModeEnum."generateWaves"  # Mode
              # "Live video for Calibration and 2D\nScan Modes.\n\nIdle Video for MultiD Scan modes\nUNTIL Begin Scan Button pressed?\n\nMultiD is waiting for trigger"
              n105 = event-data() -> ()  [unwired: 1 in, 6 out]
              n106 = Bundle("Enum"=CameraControlTypeDef."Trigger Source", "Value"=w610) -> (w611:cluster{"Enum":T8, "Value":T1})  [unwired: 1 in]
              n107 = Bundle("Mode"=w613, "Value"=w610) -> (w612:cluster{"Mode":T7, "Value":T1})  [unwired: 1 in]
              n108 = Enqueue Element(queue=w616, element=w611) -> ()  [unwired: 2 in, 3 out]
              n109 = Enqueue Element(queue=w615, element=w612) -> ()  [unwired: 2 in, 3 out]
            }
            event Value Change {
              n110 = event-data() -> ()  [unwired: 1 in, 6 out]
              n111 = Bundle("Enum"=CameraControlTypeDef."Readout Mode", "Value"=w619) -> (w618:cluster{"Enum":T8, "Value":T1})  [unwired: 1 in]
              n112 = Enqueue Element(queue=w621, element=w618) -> ()  [unwired: 2 in, 3 out]
            }
            event Value Change {
              w623 = ModeEnum."generateWaves"  # Mode
              n113 = event-data() -> ()  [unwired: 1 in, 6 out]
              n114 = Bundle("Enum"=CameraControlTypeDef."ROI", "Value"=w624) -> (w629:cluster{"Enum":T8, "Value":T1})  [unwired: 1 in]
              n115 = Bundle("Mode"=w623, "Value"=w624) -> (w626:cluster{"Mode":T7, "Value":T1})  [unwired: 1 in]
              n116 = Enqueue Element(queue=w628, element=w629) -> ()  [unwired: 2 in, 3 out]
              n117 = Enqueue Element(queue=w625, element=w626) -> ()  [unwired: 2 in, 3 out]
            }
            event Value Change {
              w633 = ModeEnum."generateWaves"  # Mode
              n118 = event-data() -> ()  [unwired: 1 in, 6 out]
              n119 = Bundle("Mode"=w633, "Value"=w631) -> (w634:cluster{"Mode":T7, "Value":T1})  [unwired: 1 in]
              n120 = Enqueue Element(queue=w632, element=w634) -> ()  [unwired: 2 in, 3 out]
            }
            event "Record": Value Change {
              n121 = event-data() -> ("NewVal"=w636:bool)  [unwired: 1 in, 5 out]
              n122 = case shown="True" w636 {
                tunnel: w638 -> [_ w643]
                tunnel: w637 -> [_ w641]
                frame False {
                }
                frame True {
                  n123 = Bundle("Enum"=CameraControlTypeDef."Ram Record", "Value"=w641) -> (w640:cluster{"Enum":T8, "Value":T1})  [unwired: 1 in]
                  n124 = Enqueue Element(queue=w643, element=w640) -> ()  [unwired: 2 in, 3 out]
                }
              }
            }
            event Value Change {
              w648 = ModeEnum."generateWaves"  # Mode
              n125 = event-data() -> ()  [unwired: 1 in, 6 out]
              n126 = Bundle("Mode"=w648, "Value"=w646) -> (w647:cluster{"Mode":T7, "Value":T1})  [unwired: 1 in]
              n127 = Enqueue Element(queue=w645, element=w647) -> ()  [unwired: 2 in, 3 out]
            }
            event Value Change {
              w655 = ModeEnum."generateWaves"  # Mode
              n128 = event-data() -> ()  [unwired: 1 in, 6 out]
              n129 = Bundle("Enum"=CameraControlTypeDef."Update", "Value"=w652) -> (w653:cluster{"Enum":T8, "Value":T1})  [unwired: 1 in]
              n130 = Bundle("Mode"=w655, "Value"=w652) -> (w654:cluster{"Mode":T7, "Value":T1})  [unwired: 1 in]
              n131 = Enqueue Element(queue=w651, element=w653) -> ()  [unwired: 2 in, 3 out]
              n132 = Enqueue Element(queue=w650, element=w654) -> ()  [unwired: 2 in, 3 out]
            }
            event "Signals Debugger": Value Change {
              n133 = event-data() -> ()  [unwired: 1 in, 6 out]
              n134 = case shown="True" "Signals Debugger" {
                frame False {
                }
                frame True {
                  n135 = vi-ref "Graph.vi"() -> (w659:refnum<vi>)
                  n136 = invoke class="VI" method="FP.Open"(reference=w659, "Activate"=TRUE ("Front Panel Window:Open"), "State"=T12."Standard") -> ()  [unwired: 2 in, 5 out]
                }
              }
            }
            event "Scan": Value Change {
              n137 = event-data() -> ("NewVal"=w663:bool)  [unwired: 1 in, 5 out]
              n138 = case shown="True" w663 {
                tunnel: w666 -> [_ w671]
                tunnel: [w667 w670] -> w665
                tunnel: w664 -> [w667 w669]
                frame False {
                }
                frame True {
                  n139 = for {
                    N: "Scans" -> [_]
                    tunnel: w671 -> [w673]
                    tunnel: [w672] -> w670
                    tunnel: w669 -> [w676]
                    w675 = ModeEnum."runWaves"  # Mode
                    n140 = Bundle("Mode"=w675, "Value"=w673) -> (w674:cluster{"Mode":T7, "Value":T1})  [unwired: 1 in]
                    n141 = Enqueue Element(queue=w676, element=w674) -> (queue out=w672:refnum<queue>)  [unwired: 2 in, 2 out]
                  }
                }
              }
            }
            event Timeout {
              n142 = event-data() -> ()  [unwired: 1 in, 3 out]
              n143 = property on="Microscope Settings" class="Clust (strict)"() -> ("Value"=w678:T1)  [unwired: 2 in, 2 out]
            }
          }
        }
        n144 = while "Camera Consumer" {
          tunnel: w159 -> [w373]
          tunnel: [w358] -> w163
          tunnel: w152 -> [w366]
          tunnel: [w374] -> w162
          shift-right: [w372] -> _
          shift-left: CameraControlTypeDef."Preview" ("Enum") -> [w362]
          tunnel: [w369] -> w157
          tunnel: w156 -> [w368]
          tunnel: w154 -> [w361]
          shift-right: [w370] -> w166
          shift-left: w167 -> [w371]
          tunnel: w141 -> [w356]
          stop <- w357 stop-if-true
          n145 = Dequeue Element(queue=w366, timeout in ms (-1)=1) -> (queue out=w365:refnum<queue>, element=w360:cluster{"Enum":T8, "Microscope Settings":T1}, timed out?=w364:bool)  [unwired: 1 in, 1 out]
          n146 = case shown="False" w364 {
            tunnel: [w376 CameraControlTypeDef."Preview" ("Enum")] -> w363
            tunnel: w362 -> [_ _]
            tunnel: w360 -> [w377 _]
            tunnel: [w375 _] -> w359
            frame False {
              n147 = Unbundle(w377) -> ("Enum"=w376:T8, "Microscope Settings"=w375:T1)
            }
            frame True {
            }
          }
          n148 = case shown="\"Ram Record\"" w363 {
            selector: w363 -> [w382 w387 w419 w438 w443 w454 w459 w464 w469 w474 w507 w525 _ w554 _]
            tunnel: w365 -> [w381 w388 w420 w439 w444 w455 w460 w465 w470 w475 _ w521 w536 w556 w575]
            tunnel: [w381 w388 w420 w439 w444 w455 w460 w465 w470 w475 _ w521 w536 w556 w575] -> w374
            tunnel: w373 -> [w383 w386 w416 w437 w442 w453 w458 w463 w468 w473 w502 w524 w528 w553 w566]
            tunnel: [w383 w386 w398 w437 w442 w453 w458 w463 w468 w473 w476 w524 w527 w553 w567] -> w358
            tunnel: [w382 w387 w419 w438 w443 w454 w459 w464 w469 w474 w507 w525 CameraControlTypeDef."Preview" ("Enum") w554 w557] -> w372
            tunnel: w371 -> [w380 w385 w400 w436 w440 w451 w457 w462 w467 w472 w504 w523 w534 w555 w569]
            tunnel: [w380 w385 w399 w436 w440 w450 w457 w462 w467 w472 w478 w523 w532 w555 w568] -> w370
            tunnel: [w379 w384 w389 w435 w441 w452 w456 w461 w466 w471 w506 w522 w530 w552 w570] -> w369
            tunnel: w368 -> [w379 w384 _ w435 w441 w452 w456 w461 w466 w471 w506 w522 w530 w552 _]
            tunnel: w361 -> [_ _ w409 _ _ _ _ _ _ _ _ _ w529 _ _]
            tunnel: w359 -> [_ _ w394 _ _ w449 _ _ _ _ w501 _ _ _ w559]
            tunnel: w356 -> [_ _ w396 _ _ _ _ _ _ _ _ _ _ _ _]
            frame "Idle" {
            }
            frame "IntervalLineInt" {
            }
            frame "Ram Record" {
              w390 = 1 items=["Snap", "Sequence"] ("Capture mode")
              w413 = 0 items=["Snap", "Sequence"] ("Capture mode")
              n149 = call "tm_stopcapture.vi"("error in (no error)"=w416, "Handle in"=w400) -> ("error out"=w417:errorcluster, "Handle out"=w418:u32)  [unwired: 8 in]
              n150 = call "tm_unpreparecapture.vi"("error in (no error)"=w417, "Handle in"=w418) -> ("error out"=w415:errorcluster, "Handle out"=w414:u32)  [unwired: 8 in]
              n151 = call "tm_preparecapture.vi"("error in (no error)"=w415, "Frames"="Frames", "Capture mode"=w413, "Handle in"=w414) -> ("error out"=w411:errorcluster, "Buffer Info"=w391:T5, "Handle out"=w412:u32)  [unwired: 4 in, 1 out]
              n152 = call "tm_startcapture_b.vi"("error in (no error)"=w411, "Handle in"=w412) -> ("error out"=w392:errorcluster, "Handle out"=w410:u32)  [unwired: 8 in]
              n153 = Bundle("Mode"=ModeEnum."runWaves", "Microscope Settings"=w394) -> (w393:cluster{"Mode":T7, "Microscope Settings":T1})  [unwired: 1 in]
              n154 = Enqueue Element(queue=w396, element=w393, error in (no error)=w392) -> ()  [unwired: 1 in, 3 out]
              n155 = for {
                N: "Frames" -> [_]
                tunnel: w392 -> [w434]
                tunnel: w410 -> [w433]
                tunnel: w409 -> [w427]
                tunnel: [w425] -> w405
                tunnel: [w424] -> w404
                tunnel: w391 -> [w423]
                n156 = call "tm_waitnextframe.vi"("error in (no error)"=w434, "Handle in"=w433) -> ("error out"=w432:errorcluster, "Handle out"=w431:u32)  [unwired: 6 in, 2 out]
                n157 = call "tm_getframe_a.vi"("error in (no error)"=w432, "Buffer Info"=w423, "Handle in"=w431) -> ("error out"=w425:errorcluster, "Data 16"=w430:u16[][], "Handle out"=w424:u32)  [unwired: 4 in, 2 out]
                n158 = Bundle By Name(cluster=T10 {"State"=enum."Start Sequence", "Stack Number"=0, "Image"=[], "Stacks"=0} ("element"), "State"=Stack_Track."Save Image", "Stack Number"=0, "Image"=w430, "Stacks"=1) -> (w426:T10)
                n159 = Enqueue Element(queue=w427, element=w426) -> ()  [unwired: 2 in, 3 out]
              }
              n160 = call "tm_stopcapture.vi"("error in (no error)"=w405, "Handle in"=w404) -> ("error out"=w406:errorcluster, "Handle out"=w403:u32)  [unwired: 8 in]
              n161 = call "tm_unpreparecapture.vi"("error in (no error)"=w406, "Handle in"=w403) -> ("error out"=w407:errorcluster, "Handle out"=w402:u32)  [unwired: 8 in]
              n162 = call "tm_preparecapture.vi"("error in (no error)"=w407, "Capture mode"=w390, "Handle in"=w402) -> ("error out"=w408:errorcluster, "Buffer Info"=w389:T5, "Handle out"=w401:u32)  [unwired: 5 in, 1 out]
              n163 = call "tm_startcapture_b.vi"("error in (no error)"=w408, "Handle in"=w401) -> ("error out"=w398:errorcluster, "Handle out"=w399:u32)  [unwired: 8 in]
            }
            frame "HardDisk Record" {
            }
            frame "Disengage Update" {
            }
            frame "Update", Default {
              w446 = u32 2049184 items=["SENSOR MODE"=4212128, "CCD MODE"=4212384, "READOUT MODE"=4211872, "ACTIVE VIEW INDEX"=4343136, "BITS PER CHANNEL"=4342976, "IMAGE PIXEL TYPE"=4343296, "BINNING"=4215968, "EXPOSURE TIME"=2049184, "CONTRAST GAIN"=3163312, "CONTRAST OFFSET"=3163328, "LIGHT MODE"=2114720, "SENSITIVITY"=2114992, "PHOTON IMAGING MODE"=2115200, "HIGH DYNAMIC RANGE MODE"=3163360, "WHITE BALANCE"=3163568, "TEMPERATURE"=2115232, "TEMPERATURE TARGET"=2115264, "SENSOR COOLER FAN"=2115296, "LINEBUNDLE HEIGHT"=4212192, "MECHANICAL SHUTTER"=2115488, "BACK FOCUS POSITION"=8422304, "TRIGGER CONNECTOR"=1066432, "TRIGGER SOURCE"=1066144, "OUTPUT TRIGGER SOURCE"=1852576, "TRIGGER GLOBAL EXPOSURE"=2049680, "FIRST TRIGGER BEHAVIOR"=2049696, "CHANNEL SYNC"=1852352, "READOUT DIRECTION"=4211904, "PRE HSYNC COUNT"=1852704, "INTERNAL LINE SPEED"=4226000, "INTERNAL LINE INTERVAL"=4226016] ("Parameter")
              n164 = Unbundle By Name(w449) -> ("Exposure/ms"=w448:dbl)  [unwired: 1 out]
              n165 = Divide(x=w448, y=1000.0) -> (x/y=w445:dbl)
              n166 = call "tm_setparameter_a.vi"("Value in"=w445, "Parameter"=w446, "Handle in"=w451) -> ("Handle out"=w450:u32)  [unwired: 7 in, 1 out]
            }
            frame "ROI" {
            }
            frame "Binning" {
            }
            frame "Scan Mode" {
            }
            frame "Trigger Mode" {
            }
            frame "Readout Mode" {
              w482 = 1 items=["Snap", "Sequence"] ("Capture mode")
              w488 = u32 4194832  # Sensor Mode
              w491 = u32 2031888  # Exposure time
              n167 = Unbundle By Name(w501) -> ("Exposure/ms"=w500:dbl, "Slit.Slit Width /%"=w496:dbl, "Slit.Scanning Mode"=w486:dbl)
              n168 = call "tm_stopcapture.vi"("error in (no error)"=w502, "Handle in"=w504) -> ("error out"=w505:errorcluster, "Handle out"=w503:u32)  [unwired: 8 in]
              n169 = Divide(x=w500, y=1000.0) -> (x/y=w498:dbl)
              n170 = Multiply(x=w496, y=2048 ("input variable")) -> (x*y=w495:dbl)
              n171 = call "tm_unpreparecapture.vi"("error in (no error)"=w505, "Handle in"=w503) -> ("error out"=w483:errorcluster, "Handle out"=w487:u32)  [unwired: 8 in]
              n172 = call "tm_setpropertyvalue.vi"("error in (no error)"=w483, "Value in"=w486, "Property ID"=w488, "Handle in"=w487) -> ("error out"=w484:errorcluster, "Handle out"=w485:u32)  [unwired: 6 in]
              n173 = Divide(x=w495, y=100.0) -> (x/y=w493:dbl)
              n174 = case shown="1, Default" w486 {
                tunnel: [w510 w511] -> w492
                tunnel: w498 -> [w510 w519]
                tunnel: w493 -> [_ w518]
                tunnel: w485 -> [w509 w513]
                tunnel: [w509 w515] -> w490
                tunnel: [w508 w514] -> w489
                tunnel: w484 -> [w508 w512]
                frame 1, Default {
                }
                frame 12 {
                  w517 = u32 4208720  # Line Interval
                  n175 = formula code="slitExpos=frameInter*LW/(LinesToReadout\n+10+LW);\nlineInter = slitExpos / LW;"("frameInter"=w519, "LW"=w518, "LinesToReadout"=2048 ("input variable")) -> ("slitExpos"=w511:dbl, "lineInter"=w516:dbl)
                  n176 = call "tm_setpropertyvalue.vi"("error in (no error)"=w512, "Value in"=w516, "Property ID"=w517, "Handle in"=w513) -> ("error out"=w514:errorcluster, "Handle out"=w515:u32)  [unwired: 6 in]
                }
              }
              n177 = call "tm_setpropertyvalue.vi"("error in (no error)"=w489, "Value in"=w492, "Property ID"=w491, "Handle in"=w490) -> ("error out"=w477:errorcluster, "Handle out"=w479:u32)  [unwired: 6 in]
              n178 = call "tm_preparecapture.vi"("error in (no error)"=w477, "Capture mode"=w482, "Handle in"=w479) -> ("error out"=w481:errorcluster, "Handle out"=w480:u32)  [unwired: 5 in, 2 out]
              n179 = call "tm_startcapture_b.vi"("error in (no error)"=w481, "Handle in"=w480) -> ("error out"=w476:errorcluster, "Handle out"=w478:u32)  [unwired: 8 in]
            }
            frame "Readout Direction" {
            }
            frame "Preview" {
              n180 = call "tm_waitnextframe.vi"("error in (no error)"=w528, "Timeout"=500, "Handle in"=w534) -> ("error out"=w526:errorcluster, "Handle out"=w533:u32)  [unwired: 5 in, 2 out]
              n181 = case shown="No Error" w526 {
                selector: w526 -> [w537 w551]
                tunnel: w533 -> [w549 w550]
                tunnel: [w548 w550] -> w532
                tunnel: w530 -> [w547 _]
                tunnel: w529 -> [w546 _]
                tunnel: w528 -> [w541 _]
                tunnel: [w538 w551] -> w527
                frame No Error {
                  w543 = 0 ("Timeout")
                  n182 = call "tm_getframe_a.vi"("error in (no error)"=w537, "Buffer Info"=w547, "Handle in"=w549) -> ("error out"=w539:errorcluster, "Data 16"=w544:u16[][], "Handle out"=w548:u32)  [unwired: 4 in, 2 out]
                  n183 = Bundle("State"=Stack_Track."Display", "Timeout"=w543, "Data 16"=w544, "Timeout"=w543) -> (w542:T15)  [unwired: 1 in]
                  n184 = Enqueue Element(queue=w546, element=w542, error in (no error)=w541) -> (error out=w540:errorcluster)  [unwired: 1 in, 2 out]
                  n185 = Merge Errors(w539, w540) -> (w538:errorcluster)
                }
                frame Error {
                }
              }
            }
            frame "ROIWindow" {
            }
            frame "Trigger Source" {
              (unwired) u32 1066144 items=["SENSOR MODE"=4212128, "CCD MODE"=4212384, "READOUT MODE"=4211872, "ACTIVE VIEW INDEX"=4343136, "BITS PER CHANNEL"=4342976, "IMAGE PIXEL TYPE"=4343296, "BINNING"=4215968, "EXPOSURE TIME"=2049184, "CONTRAST GAIN"=3163312, "CONTRAST OFFSET"=3163328, "LIGHT MODE"=2114720, "SENSITIVITY"=2114992, "PHOTON IMAGING MODE"=2115200, "HIGH DYNAMIC RANGE MODE"=3163360, "WHITE BALANCE"=3163568, "TEMPERATURE"=2115232, "TEMPERATURE TARGET"=2115264, "SENSOR COOLER FAN"=2115296, "LINEBUNDLE HEIGHT"=4212192, "MECHANICAL SHUTTER"=2115488, "BACK FOCUS POSITION"=8422304, "TRIGGER CONNECTOR"=1066432, "TRIGGER SOURCE"=1066144, "OUTPUT TRIGGER SOURCE"=1852576, "TRIGGER GLOBAL EXPOSURE"=2049680, "FIRST TRIGGER BEHAVIOR"=2049696, "CHANNEL SYNC"=1852352, "READOUT DIRECTION"=4211904, "PRE HSYNC COUNT"=1852704, "INTERNAL LINE SPEED"=4226000, "INTERNAL LINE INTERVAL"=4226016] ("Parameter")
              w565 = 1 items=["Snap", "Sequence"] ("Capture mode")
              n186 = Unbundle By Name(w559) -> ("Mode"=w558:enum16{"X", "XY", "XYZ", "XYZT", "XYZC"})
              n187 = call "tm_stopcapture.vi"("error in (no error)"=w566, "Handle in"=w569) -> ("error out"=w573:errorcluster, "Handle out"=w574:u32)  [unwired: 8 in]
              n188 = call "tm_unpreparecapture.vi"("error in (no error)"=w573, "Handle in"=w574) -> ("error out"=w561:errorcluster, "Handle out"=w564:u32)  [unwired: 8 in]
              n189 = case shown="\"XYZT\"" w558 {
                tunnel: [T9 {"Mode"=2, "Polarity"=2, "Times"=2, "Delay"=0.0} ("Parameters") T9 {"Mode"=2, "Polarity"=2, "Times"=2, "Delay"=0.0} ("Parameters") T9 {"Mode"=2, "Polarity"=2, "Times"=2, "Delay"=0.0} ("Parameters") T9 {"Mode"=1, "Polarity"=2, "Times"=2, "Delay"=0.0} ("Parameters") T9 {"Mode"=1, "Polarity"=2, "Times"=2, "Delay"=0.0} ("Parameters")] -> w562
                tunnel: [CameraControlTypeDef."Preview" ("Enum") CameraControlTypeDef."Idle" ("Enum") CameraControlTypeDef."Idle" ("Enum") CameraControlTypeDef."Idle" ("Enum") CameraControlTypeDef."Preview" ("Enum")] -> w557
                frame "XY", Default {
                }
                frame "XYZT" {
                }
                frame "XYZ" {
                }
                frame "XYZC" {
                }
                frame "X" {
                }
              }
              n190 = call <userlib>:"tm_setinputtrigger.vi"("error in (no error)"=w561, "Parameters"=w562, "Handle in"=w564) -> ("error out"=w560:errorcluster, "Handle out"=w563:u32)  [unwired: 7 in]
              n191 = call "tm_preparecapture.vi"("error in (no error)"=w560, "Capture mode"=w565, "Handle in"=w563) -> ("error out"=w572:errorcluster, "Buffer Info"=w570:T5, "Handle out"=w571:u32)  [unwired: 5 in, 1 out]
              n192 = call "tm_startcapture_b.vi"("error in (no error)"=w572, "Handle in"=w571) -> ("error out"=w567:errorcluster, "Handle out"=w568:u32)  [unwired: 8 in]
            }
          }
          n193 = local read "stop"() -> (w357:bool)
        }
        n194 = while "Tiff Consumer" {
          tunnel: [w316] -> w164
          tunnel: [w319] -> w161
          tunnel: w154 -> [w321]
          tunnel: w153 -> [w313]
          shift-right: [w311] -> _
          shift-left: _ -> [_]
          stop <- w323 stop-if-true
          # "Delay, maybe?\nCheck"
          n195 = Dequeue Element(queue=w321, timeout in ms (-1)=1) -> (queue out=w318:refnum<queue>, element=w320:T10, error out=w317:errorcluster)  [unwired: 1 in, 1 out]
          n196 = Unbundle By Name(w320) -> ("State"=w314:T11, "Image"=w315:u16[][])  [unwired: 1 out]
          n197 = case shown="\"Save Image\"" w314 {
            tunnel: [w329 w332 w334 w338 w341 w344 w347 w355] -> w319
            tunnel: w318 -> [w329 w332 w334 w338 w341 w344 w347 w355]
            tunnel: w315 -> [w325 _ _ _ _ _ _ w354]
            tunnel: w313 -> [w328 w330 w333 w336 w339 w342 w345 w352]
            tunnel: w317 -> [w327 w331 w335 w337 w340 w343 w346 w353]
            tunnel: [w326 w331 w335 w337 w340 w343 w346 w351] -> w316
            tunnel: [w324 w330 w333 w336 w339 w342 w345 w348] -> w311
            frame "Display" {
              n198 = call "IMAQ ArrayToImage"("Image Pixels (U16)"=w325, "error in (no error)"=w327, "Image"=w328) -> ("error out"=w326:errorcluster, "Image Out"=w324:T3)  [unwired: 7 in]
            }
            frame "Idle", Default {
            }
            frame "Start Sequence" {
            }
            frame "Read Disk" {
            }
            frame "STOP" {
            }
            frame "Collecting" {
            }
            frame "End" {
            }
            frame "Save Image" {
              n199 = call "4Digit File Incrementer.vi"("path"="Imaging Folder") -> ("appended path"=w349:path)  [unwired: 10 in]
              "appended path" <- w349
              n200 = call "IMAQ ArrayToImage"("Image Pixels (U16)"=w354, "error in (no error)"=w353, "Image"=w352) -> ("error out"=w351:errorcluster, "Image Out"=w348:T3)  [unwired: 7 in]
              n201 = local write "Imaging Folder"(w349) -> ()
              n202 = call-poly "IMAQ Write File 2"("File Path"=w349, "Image"=w348) -> ()  [unwired: 8 in, 2 out]
            }
          }
          "Image" <- w311
          n203 = call "IMAQ Histograph"("Image"=w311) -> ("Histogram Graph"=→"Histogram":T4)  [unwired: 7 in, 3 out]
          n204 = local read "stop"() -> (w323:bool)
        }
        n205 = Merge Errors(w163, w164, w143) -> (w165:errorcluster)
      }
      frame "deinit" {
        n206 = call <vilib>:"DAQmx Stop Task.vi"("task/channels in"=w689) -> ("task out"=w690:refnum<k21>)  [unwired: 13 in, 1 out]
        n207 = call <vilib>:"DAQmx Stop Task.vi"("task/channels in"=w691) -> ("task out"=w692:refnum<k21>)  [unwired: 13 in, 1 out]
        n208 = call <vilib>:"DAQmx Clear Task.vi"("task in"=w690) -> ("error out"=w686:errorcluster)  [unwired: 14 in]
        n209 = call "tm_stopcapture.vi"("error in (no error)"=w701, "Handle in"=w697) -> ("error out"=w704:errorcluster, "Handle out"=w703:u32)  [unwired: 8 in]
        n210 = call <vilib>:"DAQmx Clear Task.vi"("task in"=w692) -> ("error out"=w687:errorcluster)  [unwired: 14 in]
        n211 = call "tm_unpreparecapture.vi"("error in (no error)"=w704, "Handle in"=w703) -> ("error out"=w705:errorcluster, "Handle out"=w702:u32)  [unwired: 8 in]
        n212 = call "tm_closecamera.vi"("error in (no error)"=w705, "Handle in"=w702) -> ("error out"=w706:errorcluster)  [unwired: 9 in]
        n213 = Flush Queue(queue=w679) -> (queue out=w685:refnum<queue>)  [unwired: 1 in, 2 out]
        n214 = call "tm_deinitialize.vi"("error in (no error)"=w706) -> ("error out"=w682:errorcluster)  [unwired: 10 in]
        n215 = Release Queue(queue=w680, error in (no error)=w682) -> (error out=w699:errorcluster)  [unwired: 1 in, 2 out]
        n216 = Release Queue(queue=w685) -> (error out=w688:errorcluster)  [unwired: 2 in, 2 out]
        n217 = Flush Queue(queue=w684, error in (no error)=w682) -> (queue out=w683:refnum<queue>, error out=w681:errorcluster)  [unwired: 1 out]
        n218 = Release Queue(queue=w683, error in (no error)=w681) -> (error out=w698:errorcluster)  [unwired: 1 in, 2 out]
        n219 = Merge Errors(w699, w698, w688, w687, w686) -> (w700:errorcluster)
      }
    }
    n220 = Or(x="stop", y=w17) -> (x .or. y?=w18:bool)
  }
  "error IO" <- w5
  n221 = disable-structure shown="Enabled" {
    frame Disabled {
      # "Parallise decode buffer"
      n222 = call "tm_startcapture_b.vi"() -> ()  [unwired: 10 in, 2 out]
      n223 = call "tm_waitnextframe.vi"() -> ()  [unwired: 8 in, 4 out]
      n224 = call "tm_getframe_a.vi"() -> ()  [unwired: 7 in, 5 out]
    }
    frame Enabled {
    }
  }
